vi "Adjust_VI_Properties.vi"(6 "VI refnum in":refnum<vi>, 8 "error in (no error)":errorcluster, 9 "sourceInclusion":T3, 10 "properties in":T1[](array[typedef]), 11 "AB_Application in":refnum<class "AB_Application.lvclass">) -> (0 "error out":errorcluster, 1 "defaultSaveLevel":u32, 2 "properties out":T1[](array[typedef]), 3 "AB_Application out":refnum<class "AB_Application.lvclass">)   [LabVIEW 2020, in "AB_Application.lvclass"]
uses:
  <vilib>/AppBuilder/AB_Classes/Application/AB_Application.lvclass
  <vilib>/AppBuilder/AB_Source_Properties.ctl
  <vilib>/AppBuilder/AB_Source_Property_Type.ctl
  e:/builds/penguin/labview/branches/2020/dev/dist/vi.lib/AppBuilder/AB_Classes/TargetFile/AB_Targetfile.lvclass
  <vilib>/AppBuilder/AB_Source_Inclusion.ctl
  <vilib>/AppBuilder/AB_Classes/TargetFile/AB_Targetfile.lvclass
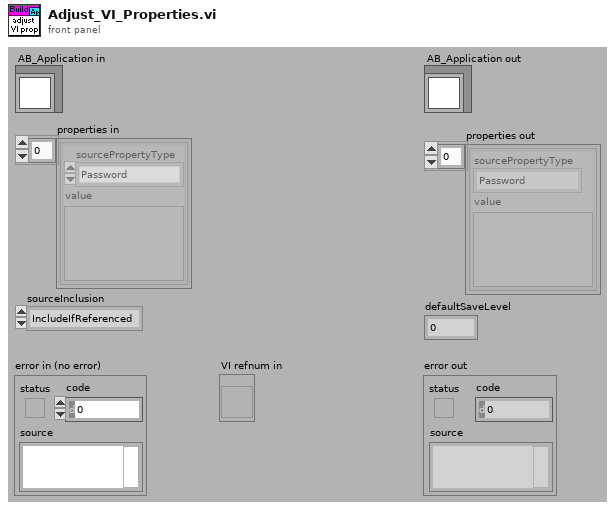
[diagram p1: front panel]
types:
  T1 = typedef "AB_Source_Properties.ctl" = cluster{"sourcePropertyType":T2, "value":variant}
  T2 = typedef "AB_Source_Property_Type.ctl" = enum16{"Remove block diagram", "Remove front panel", "Password", "Window has title bar", "Show menu bar", "Show vertical scroll bar", "Show horizontal scroll bar", "Show toolbar", "Show Abort button", "Show fp when called", "Window behavior", "Allow user to close window", "Window run-time position", "Run when opened", "Allow debugging", "Auto error handling", "Generate guard code", "Use stack variables", "Expression folding", "Integer only", "Inline subVI"}
  T3 = typedef "AB_Source_Inclusion.ctl" = enum16{"IncludeIfReferenced", "Include", "Exclude", "TopLevel"}
  T4 = typedef "AB_Targetfile.ctl" = cluster{"targetfileName":string, "targetfileGUID":string, "enableDebugging":bool, "versionInfo":cluster{"productName":string, "legalCopyright":string, "companyName":string, "internalName":string, "fileDescription":string}, "eng_consolidatedTypeInfo":string, "fastFileFormat":bool, "eng_LEIFBuildData":u32, "versionIndependent":bool}
  T5 = enum16{"Share clones between instances", "Preallocate clone for each instance"}
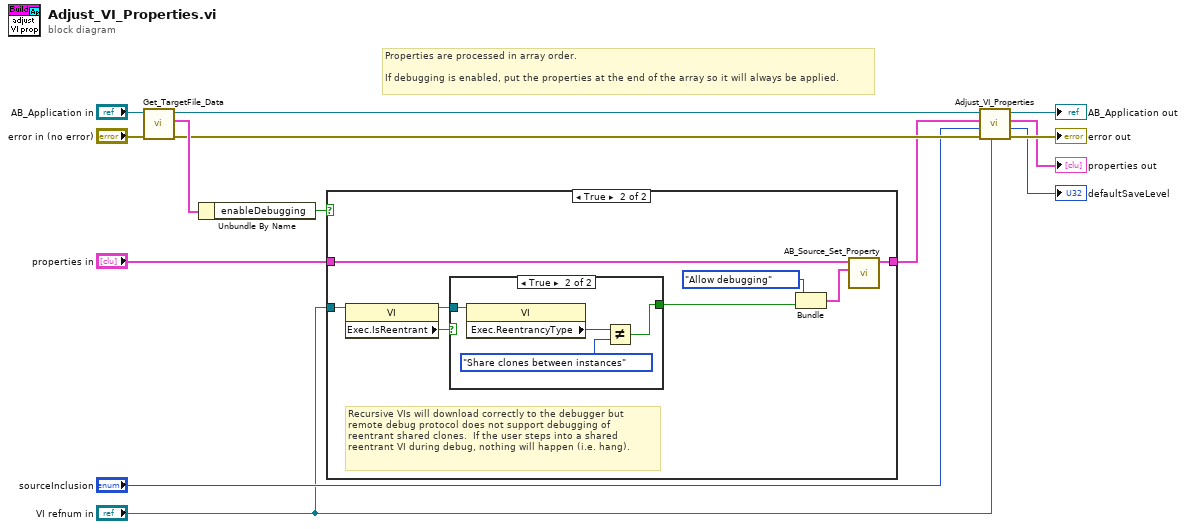
[diagram p0: block diagram]
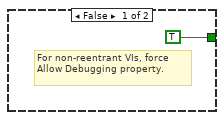
[diagram p3: hidden frame]
diagram:
  # "Properties are processed in array order.\n\nIf debugging is enabled, put the properties at the end of the array so it will always be applied."
  n1 = call <vilib>:"Get_TargetFile_Data.vi"("error in (no error)"="error in (no error)", "AB_Targetfile in"="AB_Application in") -> ("error out"=w10:errorcluster, "data"=w12:T4, "AB_Targetfile out"=w9:refnum<class "AB_Application.lvclass">)  [unwired: 7 in]
  n2 = Unbundle By Name(w12) -> ("enableDebugging"=w13:bool)
  n3 = case shown="True" w13 {
    tunnel: "properties in" -> [w15 w22]
    tunnel: [w15 w16] -> w4
    tunnel: "VI refnum in" -> [_ w20]
    frame False {
    }
    frame True {
      # "Recursive VIs will download correctly to the debugger but remote debug protocol does not support debugging of reentrant shared clones.  If the user steps into a shared reentrant VI during debug, nothing will happen (i.e. hang)."
      n4 = property class="VI"(reference=w20) -> (reference out=w17:refnum<vi>, "Exec.IsReentrant"=w19:bool)  [unwired: 1 in, 1 out]
      n5 = case shown="True" w19 {
        tunnel: [TRUE w27] -> w18
        tunnel: w17 -> [_ w28]
        frame False {
          # "For non-reentrant VIs, force Allow Debugging property."
        }
        frame True {
          n6 = property class="VI"(reference=w28) -> ("Exec.ReentrancyType"=w26:T5)  [unwired: 1 in, 2 out]
          n7 = Not Equal?(x=w26, y=T5."Share clones between instances" ("Execution:Reentrancy Type")) -> (x != y?=w27:bool)
        }
      }
      n8 = Bundle("sourcePropertyType"=AB_Source_Property_Type."Allow debugging", w18) -> (w21:cluster{"sourcePropertyType":T2, bool})  [unwired: 1 out]
      n9 = call <vilib>:"AB_Source_Set_Property.vi"("sourceProperty"=w21, "sourceProperties in"=w22) -> ("sourceProperties out"=w16:T1[])  [unwired: 1 in, 8 out]
    }
  }
  n10 = call-parent "Adjust_VI_Properties.vi"("VI refnum in"="VI refnum in", "error in (no error)"=w10, "sourceInclusion"="sourceInclusion", "properties in"=w4, "AB_Targetfile in"=w9) -> ("error out"=→"error out":errorcluster, "defaultSaveLevel"=→"defaultSaveLevel":u32, "properties out"=→"properties out":T1[], "AB_Targetfile out"=→"AB_Application out":refnum<class "AB_Application.lvclass">)  [unwired: 3 in]
